vi "Some VI 2.vi"(8 "Error In":errorcluster) -> (0 "Error Out":errorcluster, 2 "signal out 2":waveform(dbl))   [LabVIEW 2014]
uses:
  <vilib>/measure/NI_MABase.lvlib
panel:
  out "signal out":waveform(dbl)
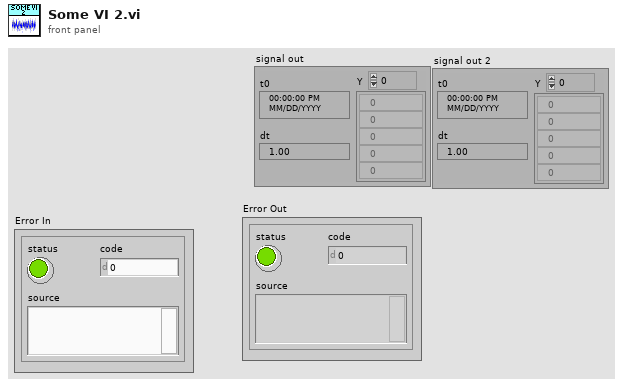
[diagram p1: front panel]
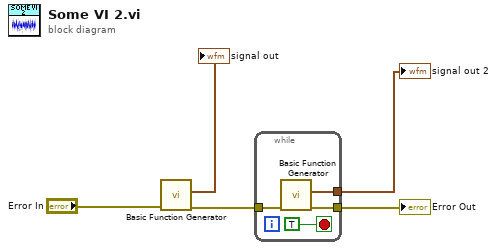
[diagram p0: block diagram]
diagram:
  n1 = call <vilib>:"Basic Function Generator.vi"("error in (no error)"="Error In") -> ("error out"=w4:errorcluster, "signal out"=→"signal out":waveform(dbl))  [unwired: 8 in, 1 out]
  n2 = while {
    tunnel: [w7] -> w1
    tunnel: w4 -> [w9]
    tunnel: [w8] -> w3
    stop <- TRUE stop-if-true
    n3 = call <vilib>:"Basic Function Generator.vi"("error in (no error)"=w9) -> ("error out"=w8:errorcluster, "signal out"=w7:waveform(dbl))  [unwired: 8 in, 1 out]
  }
  "Error Out" <- w3
  "signal out 2" <- w1
